vi "Trapezoidal Set RPM.vi"(8 "Desired RPM":dbl, 9 "Current RPM":dbl, 11 "Spinning Wheels?":bool) -> (2 "Stage 1 Time":dbl, 3 "RPM":dbl, 5 "Shooter Ready?":bool)   [LabVIEW 2015]
uses:
  Trapezoidal Motion State.ctl
  Common Code/Change Detect Double.vi
  Common Code/Change Detect Boolean.vi
  Robot Code/Robot Global Data.vi
panel:
  out "Current State":T1
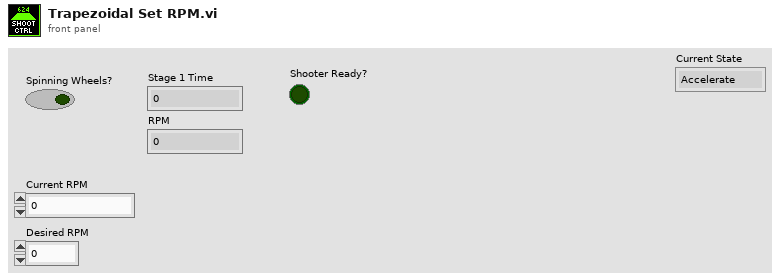
[diagram p1: front panel]
types:
  T1 = typedef "Trapezoidal Motion State.ctl" = enum16{"Accelerate", "Cruise", "Decelerate", "Finish"}
  T2 = typedef "Dashboard Control Data.ctl" = cluster{"Shooter Presets":T3, "Encoder Control":T5, "Steer PID output":cluster{"output high":dbl, "output low":dbl}, " Steer PID gains":cluster{"proportional gain (Kc)":dbl, "integral time (Ti, min)":dbl, "derivative time (Td, min)":dbl}, "Drivetrain Settings":T6, "Vision Packet":T7, "Dashboard Drivetrain Command":T8, "Info/Command Cluster":T10, "Ball Vision Packet":T11, "Intake Presets":T13, "Intake Encoder Control":T15, "Climb Presets":T16, "Goal Output Range":cluster{"output high":dbl, "output low":dbl}, "Enabled Systems":T17, "Auton Presets":T18, "Pressure M":dbl, "Pressure B":dbl, "Vision Timeout":dbl, "Auto-Shift":T19}
  T3 = typedef "Shooter Presets.ctl" = cluster{"Batter Shot":T4, "Deep Middle":T4, "Manual Shot":T4, "Left Ticks Per Rotation":dbl, "Right Ticks Per Rotation":dbl, "Low Bar Shot":T4, "Shooter RPM Tolerance":dbl, "Trigger Power":dbl, "Fire from Load Delay":i32, "Max Angle":dbl, "Min Angle":dbl, "Angle PID gains":cluster{"P":dbl, "I":dbl, "D":dbl}, "Angle Output":cluster{"output high":dbl, "output low":dbl}, "Shooter Angle Tolerance":dbl, "Vision Shoot x^2":dbl, "Vision Shoot x":dbl, "Feed Forward Max Accel":dbl, "Feed Forward Kv":dbl, "Backwards Trigger":dbl, "Shot Finish Delay (ms)":dbl, "Angle Max Current":dbl, "Angle Current Trip Time":dbl, "Intake Angle":dbl, "Vision Shoot c":dbl, "Reset?":bool, "Button Release Delay":dbl, "Angle Pot x":dbl, "Angle Pot c":dbl, "Ignore Angle?":bool, "Max RPM":dbl, "Safty Frist Angle":dbl, "Intake Danger Height":dbl, "Angle Pot B":i32, "Angle Pot M":dbl, "FF Finish RPM":dbl, "RPM PID Right":cluster{"P":dbl, "I":dbl, "D":dbl, "FF":dbl}, "RPM PID Left":cluster{"P":dbl, "I":dbl, "D":dbl, "FF":dbl}, "Backwards RPM":dbl, "Vision RPM":dbl, "Run Wheels Backward Delay":u32, "Cleat Shot":T4, "Vision Far RPM":dbl, "Vision Far Distance":dbl, "Vision Far Angle":dbl}
  T4 = typedef "Shot Presets.ctl" = cluster{"L":dbl, "R":dbl, "A":dbl}
  T5 = typedef "Encoder Control.ctl" = cluster{"Right Tick Constant":dbl, "Left Tick Constant":dbl, "Reset?":bool, "Y Dist":cluster{"PID gains":cluster{"proportional gain (Kc)":dbl, "integral time (Ti, min)":dbl, "derivative time (Td, min)":dbl}}, "Y Stop Thresh":dbl, "Y Stop Speed":dbl}
  T6 = typedef "Drivetrain Settings.ctl" = cluster{"Gyro Tolerance":dbl, "Throttle Ramp (ms)":dbl, "Kv":dbl, "Ka":dbl, "Feed Forward P":dbl, "Feed Forward D":dbl, "Goal Vision PID gains":cluster{"proportional gain (Kc)":dbl, "integral time (Ti, min)":dbl, "derivative time (Td, min)":dbl}, "Goal Detection Window":dbl, "Creep Rate":dbl, "Vision Throttle Threshold":dbl, "Min Turn Output":dbl, "Left Batter Angle":dbl, "Right Batter Angle":dbl}
  T7 = typedef "Goal Vision Packet.ctl" = cluster{"Distance":dbl, "Center X":dbl, "Center Y":dbl, "Found Target?":bool, "Robot Center":dbl, "Angle":dbl}
  T8 = typedef "Dashboard Drivetrain Command.ctl" = cluster{"Drivetrain Vision":T9}
  T9 = typedef "Drivetrain Vision.ctl" = cluster{"Goal Window":dbl, "Ball Window":dbl}
  T10 = typedef "Ball Tracking Command Cluster.ctl" = cluster{"Distance to Ball":dbl, "Desired Angle":dbl, "Command":enum16{"Turn to Ball", "Turn to Angle", "Get Distance"}, "Pixels from Center":dbl}
  T11 = typedef "Ball Vision Packet.ctl" = cluster{"Ball Detected?":bool, "Distance to Ball":dbl, "Desired Angle":dbl, "Pixels from Center":dbl, "Tracking mode":T12}
  T12 = typedef "Tracking Mode.ctl" = enum16{"Turn to Ball", "Turn to Angle"}
  T13 = typedef "Intake Presets.ctl" = cluster{"Intake Speed":dbl, "Outake Speed":dbl, "Low Height":dbl, "Half Height":dbl, "High Idle Height":dbl, "Angle Speed":dbl, "Angle Tolerance":dbl, "Encoder Scale":dbl, "Load Height":dbl, "Output Range":T14, "Rotation Power Max/Min":dbl, "MaxCurrent":dbl, "Intake Trip Time":dbl, "Idle Height":dbl, "Max Height":dbl, "Reset Encoders?":bool, "PID gains":cluster{"proportional gain (Kc)":dbl, "integral time (Ti, min)":dbl, "derivative time (Td, min)":dbl}, "Intake Stop Delay":u32, "Settle Time":dbl, "Settle Wait Time":dbl, "Pull Up Delay":dbl}
  T14 = typedef "Drivetrain Output Range.ctl" = cluster{"output high":dbl, "output low":dbl}
  T15 = typedef "IntakeEcoderControl.ctl" = cluster{"Arm Tick Constant":dbl, "Reset?":bool, "Y Dist":cluster{"PID gains":cluster{"proportional gain (Kc)":dbl, "integral time (Ti, min)":dbl, "derivative time (Td, min)":dbl}}, "Y Stop Thresh":dbl, "Y Stop Speed":dbl}
  T16 = typedef "Climb Presets.ctl" = cluster{"Pull Power":dbl, "Extend Power":dbl}
  T17 = typedef "Enabled Systems.ctl" = cluster{"Shoot":bool, "Intake":bool, "DT":bool, "Gyro":bool, "100ms":bool, "US":bool}
  T18 = typedef "Autonomous Presets.ctl" = cluster{"Pitch Limit":dbl, "Roll Limit":dbl, "Start Position":dbl, "Cross Position":dbl}
  T19 = typedef "Auto Shift Cluster.ctl" = cluster{"Delay":dbl, "Speed Thresh":dbl, "Upshift Accel":dbl, "Upshift Throttle":dbl, "Upshift Throttle Accel":dbl, "Downshift Throttle":dbl, "Downshift Throttle Accel":dbl, "Pressure Threshold":dbl}
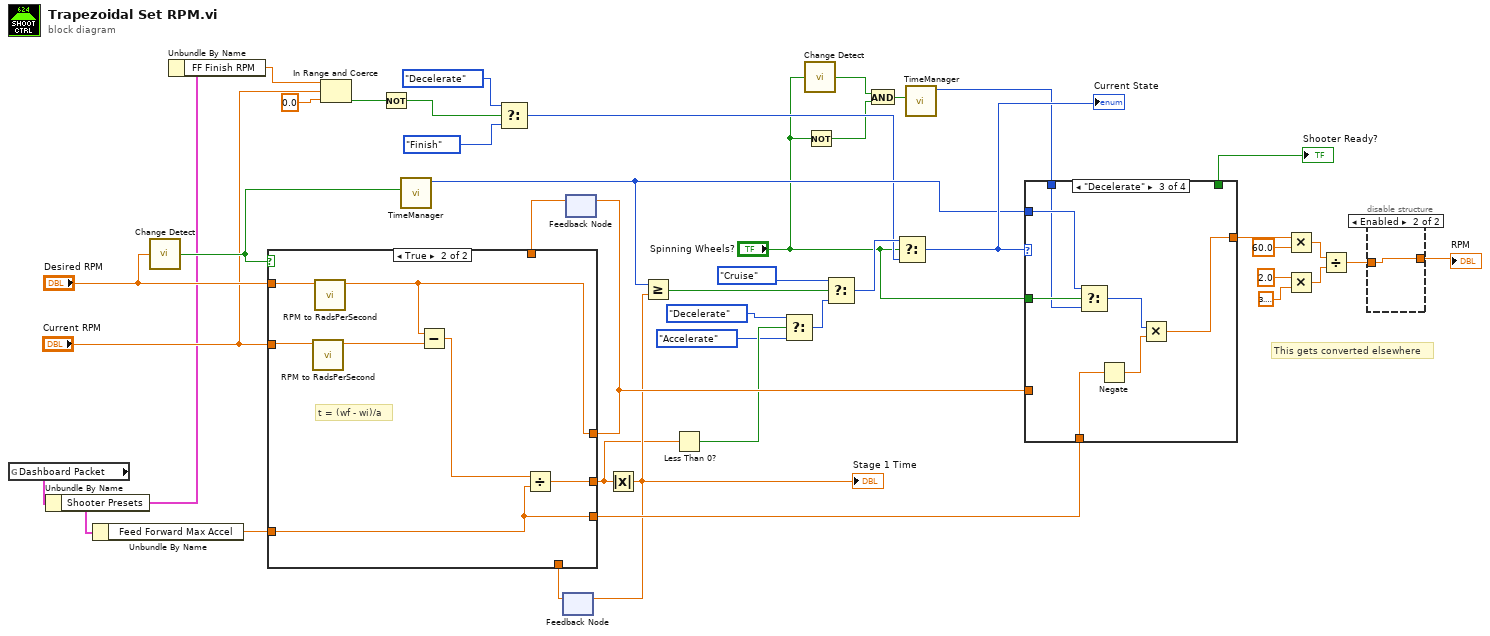
[diagram p0: block diagram]
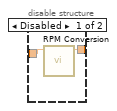
[diagram p2: hidden frame]
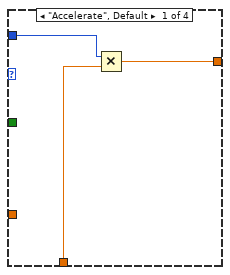
[diagram p3: hidden frame]
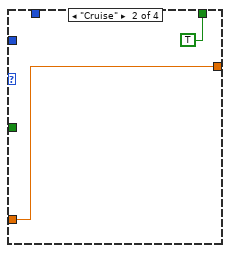
[diagram p4: hidden frame]
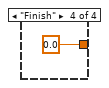
[diagram p5: hidden frame]
diagram:
  # "This gets converted elsewhere"
  n1 = global read "Robot Global Data.vi" "Dashboard Packet"() -> (w26:T2)
  n2 = Unbundle By Name(w26) -> ("Shooter Presets"=w6:T3)
  n3 = Unbundle By Name(w6) -> ("Feed Forward Max Accel"=w25:dbl)
  n4 = call-poly "Change Detect.vi"("In"="Desired RPM") -> ("Changed?"=w9:bool)
  n5 = Unbundle By Name(w6) -> ("FF Finish RPM"=w5:dbl)
  n6 = In Range and Coerce(upper limit=w5, x="Current RPM", lower limit=0.0) -> (In Range?=w4:bool)  [unwired: 1 out]
  n7 = Not(x=w4) -> (.not. x?=w3:bool)
  n8 = call "TimeManager.vi"("Reset?"=w9) -> ("Time Since Reset"=w36:u32)  [unwired: 9 in, 1 out]
  n9 = Select(t=Trapezoidal_Motion_State."Decelerate" ("Enum"), s=w3, f=Trapezoidal_Motion_State."Finish" ("Enum")) -> (s? t:f=w16:T1)
  n10 = feedback #1() -> (w41:dbl)  [unwired: 1 in]
  n11 = feedback #2() -> (w28:dbl)  [unwired: 1 in]
  n12 = case shown="True" w9 {
    tunnel: [w45 w52] -> w23
    tunnel: "Current RPM" -> [_ w49]
    tunnel: "Desired RPM" -> [_ w50]
    tunnel: w41 -> [w45 _]
    tunnel: [w43 w51] -> w35
    tunnel: [w44 w46] -> w27
    tunnel: w28 -> [w44 _]
    tunnel: w25 -> [w43 w51]
    frame False {
    }
    frame True {
      # "t = (wf - wi)/a"
      n13 = call "RPM to RadsPerSecond.vi"("Desired RPM"=w49) -> ("Numeric"=w48:dbl)  [unwired: 10 in]
      n14 = call "RPM to RadsPerSecond.vi"("Desired RPM"=w50) -> ("Numeric"=w46:dbl)  [unwired: 10 in]
      n15 = Subtract(x=w46, y=w48) -> (x-y=w47:dbl)
      n16 = Divide(x=w47, y=w51) -> (x/y=w52:dbl)
    }
  }
  n17 = feedback-in #2(w27) -> ()
  n18 = Absolute Value(x=w23) -> (abs(x)=w24:dbl)
  "Stage 1 Time" <- w24
  n19 = feedback-in #1(w24) -> ()
  n20 = Greater Or Equal?(x=w36, y=w24) -> (x >= y?=w40:bool)
  n21 = Less Than 0?(x=w23) -> (x < 0?=w22:bool)
  n22 = Select(t=Trapezoidal_Motion_State."Decelerate" ("Enum"), s=w22, f=Trapezoidal_Motion_State."Accelerate") -> (s? t:f=w19:T1)
  n23 = call-poly "Change Detect.vi"("In"="Spinning Wheels?") -> ("Changed?"=w15:bool)
  n24 = Not(x="Spinning Wheels?") -> (.not. x?=w14:bool)
  n25 = Select(t=Trapezoidal_Motion_State."Cruise" ("Enum"), s=w40, f=w19) -> (s? t:f=w38:T1)
  n26 = And(x=w15, y=w14) -> (x .and. y?=w13:bool)
  n27 = Select(t=w38, s="Spinning Wheels?", f=w16) -> (s? t:f=w37:T1)
  "Current State" <- w37
  n28 = call "TimeManager.vi"("Reset?"=w13) -> ("Time Since Reset"=w11:u32)  [unwired: 9 in, 1 out]
  n29 = case shown="\"Decelerate\"" w37 {
    tunnel: w36 -> [w55 _ w62 _]
    tunnel: w35 -> [w53 _ w64 _]
    tunnel: [w54 w57 w59 0.0] -> w34
    tunnel: w27 -> [_ w57 _ _]
    tunnel: "Spinning Wheels?" -> [_ _ w63 _]
    tunnel: w11 -> [_ _ w58 _]
    tunnel: [_ TRUE _ _] -> w10
    frame "Accelerate", Default {
      n30 = Multiply(x=w55, y=w53) -> (x*y=w54:dbl)
    }
    frame "Cruise" {
    }
    frame "Decelerate" {
      n31 = Select(t=w62, s=w63, f=w58) -> (s? t:f=w61:u32)
      n32 = Negate(x=w64) -> (-x=w60:dbl)
      n33 = Multiply(x=w61, y=w60) -> (x*y=w59:dbl)
    }
    frame "Finish" {
    }
  }
  "Shooter Ready?" <- w10
  n34 = Multiply(x=w34, y=60.0) -> (x*y=w30:dbl)
  n35 = Multiply(x=2.0, y=3.141592653589793) -> (x*y=w29:dbl)
  n36 = Divide(x=w30, y=w29) -> (x/y=w2:dbl)
  n37 = disable-structure shown="Enabled" {
    disable-tunnel: w2 -> [w67 w68]
    disable-tunnel: [w66 w68] -> w1
    frame Disabled {
      n38 = call "RPM Conversion.vi"("RPM"=w67) -> ("RPM Out"=w66:dbl)  [unwired: 10 in]
    }
    frame Enabled {
    }
  }
  "RPM" <- w1
